vi "Create.vi"   [LabVIEW 2021]
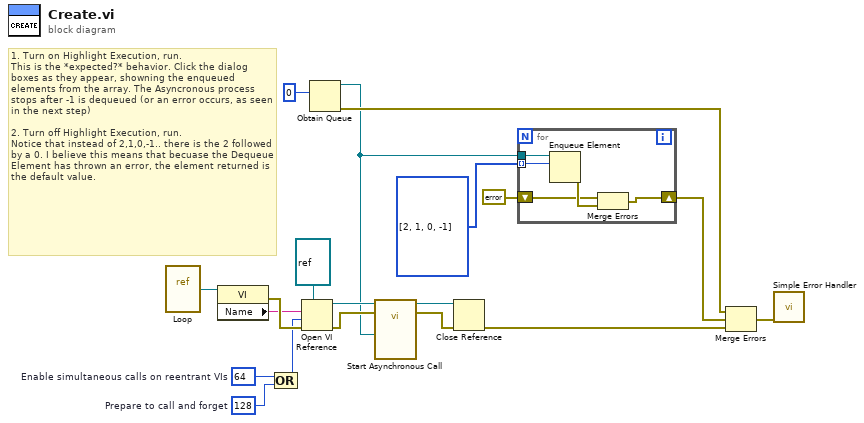
[diagram p0: block diagram]
diagram:
  w11 = 128  # Prepare to call and forget
  w12 = 64  # Enable simultaneous calls on reentrant VIs
  # "1. Turn on Highlight Execution, run.\nThis is the *expected?* behavior. Click the dialog boxes as they appear, showning the enqueued elements from the array. The Asyncronous process stops after -1 is dequeued (or an error occurs, as seen in the next step)\n\n2. Turn off Highlight Execution, run.\nNotice that instead of 2,1,0,-1.. there is the 2 followed by a 0. I believe this means that becuase the Dequeue Element has thrown an error, the element returned is the default value."
  n1 = vi-ref "Loop.vi"() -> (w15:refnum<vi>)
  n2 = property class="VI"(reference=w15) -> (error out=w14:errorcluster, "Name"=w13:string)  [unwired: 1 in, 1 out]
  n3 = Compound Arithmetic op=OR(w12, w11) -> (w10:i32)
  n4 = Open VI Reference(type specifier VI Refnum (for type only)=refnum<vi> refnum, vi path=w13, options=w10, error in (no error)=w14) -> (vi reference=w8:refnum<vi>, error out=w9:errorcluster)  [unwired: 2 in]
  n5 = Obtain Queue(element data type=0 ("I32")) -> (queue out=w4:refnum<queue>, error out=w7:errorcluster)  [unwired: 4 in, 1 out]
  n6 = call-by-ref "Start Asynchronous Call"(reference=w8, error in=w9, "Queue"=w4) -> (reference out=w1:refnum<vi>, error out=w3:errorcluster)  [unwired: 11 in]
  n7 = Close Reference(reference=w1, error in (no error)=w3) -> (error out=w2:errorcluster)
  n8 = for {
    tunnel: w4 -> [w20]
    tunnel: i32[] [2, 1, 0, -1] ("reversed array") -> [w24] mode=indexing
    shift-right: [w22] -> w18
    shift-left: errorcluster {"status"=FALSE, "code"=0, "source"=""} ("error out") -> [w21]
    n9 = Enqueue Element(queue=w20, element=w24) -> (error out=w23:errorcluster)  [unwired: 2 in, 2 out]
    n10 = Merge Errors(w21, w23) -> (w22:errorcluster)
  }
  n11 = Merge Errors(w7, w18, w2) -> (w17:errorcluster)
  n12 = call <vilib>:"Simple Error Handler.vi"("error in (no error)"=w17) -> ()  [unwired: 4 in, 5 out]
